vi "DriveRawToPosition&Velocity.vi"(8 "Velocity (Raw Sensor Units per 100 ms) B":i32, 9 "Position (Raw Sensor Units) B":i32, 10 "Velocity (Raw Sensor Units per 100 ms) A":i32, 11 "Position (Raw Sensor Units) A":i32) -> (0 "Velocity":dbl, 3 "Position":dbl)   [LabVIEW 2019]
panel:
  in  "gear ratio":dbl=11.25 format="%#_13g"
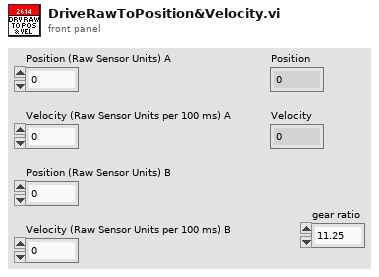
[diagram p1: front panel]
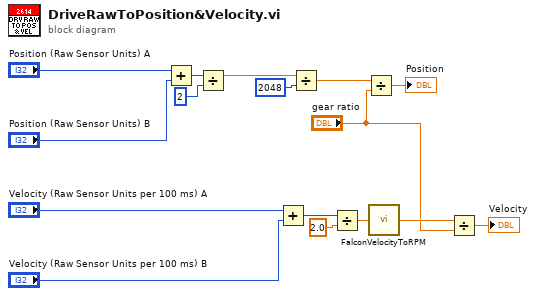
[diagram p0: block diagram]
diagram:
  n1 = Add(x="Position (Raw Sensor Units) A", y="Position (Raw Sensor Units) B") -> (x+y=w14:i32)
  n2 = Divide(x=w14, y=2) -> (x/y=w2:dbl)
  n3 = Add(x="Velocity (Raw Sensor Units per 100 ms) A", y="Velocity (Raw Sensor Units per 100 ms) B") -> (x+y=w6:i32)
  n4 = Divide(x=w2, y=2048) -> (x/y=w11:dbl)
  n5 = Divide(x=w6, y=2.0) -> (x/y=w8:dbl)
  n6 = Divide(x=w11, y="gear ratio") -> (x/y=→"Position":dbl)
  n7 = call "FalconVelocityToRPM.vi"("raw sensor units / 100 ms"=w8) -> ("RPM"=w9:dbl)  [unwired: 4 in]
  n8 = Divide(x=w9, y="gear ratio") -> (x/y=→"Velocity":dbl)
